vi "Controller Orbit Correction Algorithm.vi"(0 "FOFB Variables":T1, 1 "Corrector Kick Vector in":dbl[](array[numeric]), 2 "Beam Position Vector":dbl[](array[numeric]), 3 "Active?":bool, 5 "error in (no error)":errorcluster, 8 "Corrector Kick Vector Manual Setpoint in":dbl[](array[numeric])) -> (14 "Good value?":bool=TRUE, 15 "Corrector Kick Vector out":dbl[](array[numeric]), 19 "error out":errorcluster)   [LabVIEW 2011, in "Controller VIs.lvlib"]
doc: "Computes the correction algorithm to the selected BPM readings and returns the calculated corrector kick vector to be applied to the FOFB actuators."
uses:
  Controller VIs.lvlib
  Types Definitions/Type FOFB Variables.ctl
  Common VIs.lvlib
  Type Definitions.lvlib
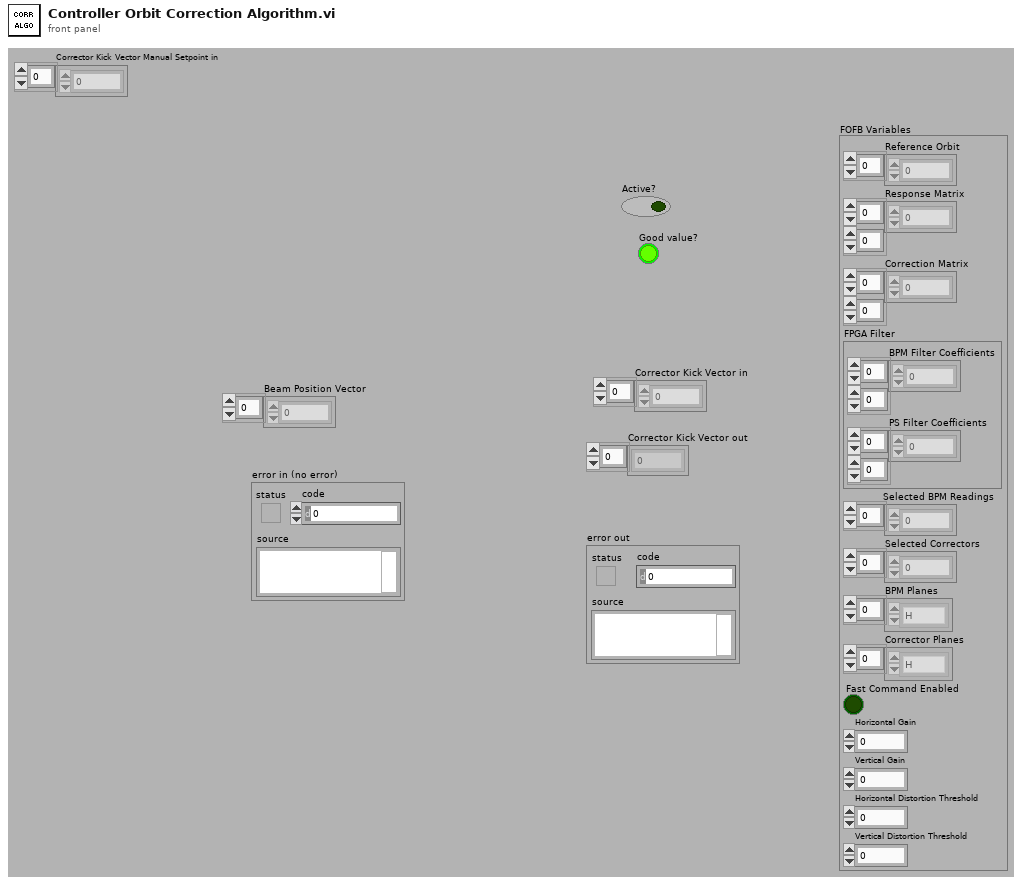
[diagram p1: front panel]
types:
  T1 = typedef "Type Definitions.lvlib/Type FOFB Variables.ctl" = cluster{"Reference Orbit":dbl[], "Response Matrix":dbl[][], "Correction Matrix":dbl[][], "FPGA Filter":cluster{"BPM Filter Coefficients":dbl[][], "PS Filter Coefficients":dbl[][]}, "Selected BPM Readings":u32[], "Selected Correctors":u32[], "BPM Planes":enum8{"H", "V"}[], "Corrector Planes":enum8{"H", "V"}[], "Fast Command Enabled":bool, "Horizontal Gain":dbl, "Vertical Gain":dbl, "Horizontal Distortion Threshold":dbl, "Vertical Distortion Threshold":dbl}
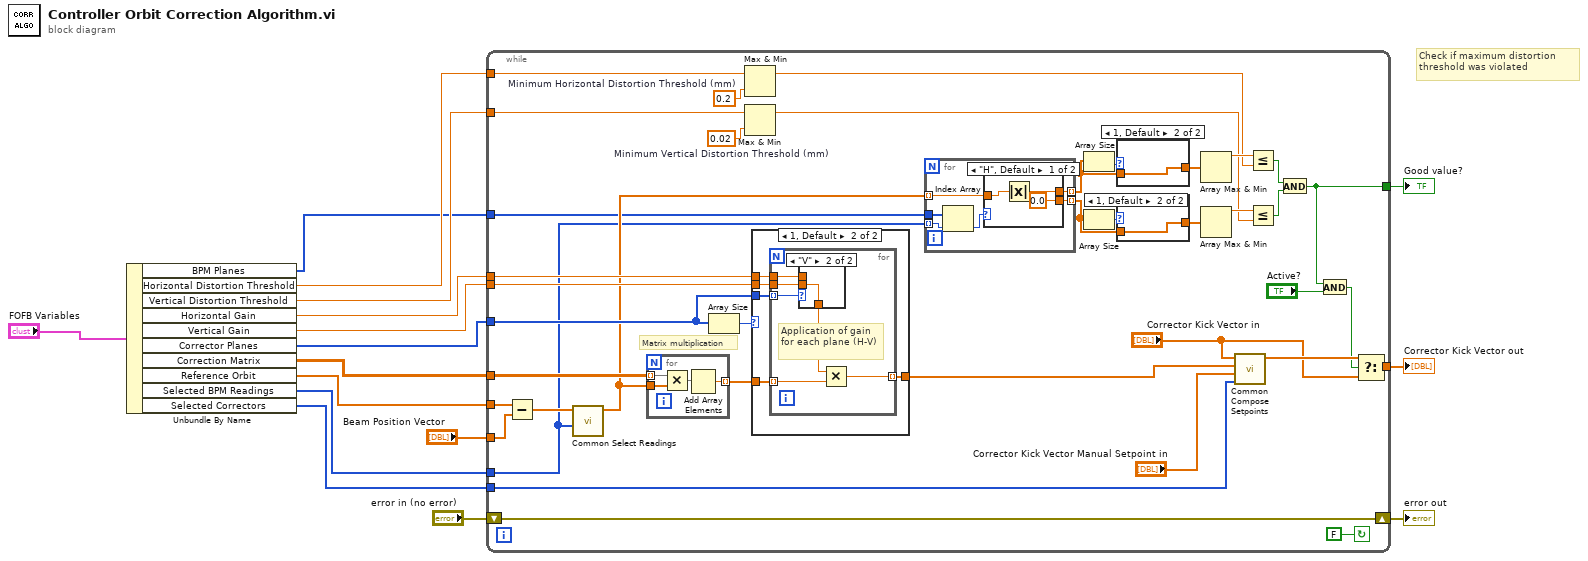
[diagram p0: block diagram]
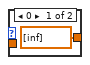
[diagram p2: hidden frame]
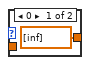
[diagram p3: hidden frame]
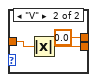
[diagram p4: hidden frame]
diagram:
  # "Check if maximum distortion threshold was violated"
  n1 = Unbundle By Name("FOFB Variables") -> ("BPM Planes"=w1:enum8{"H", "V"}[], "Horizontal Distortion Threshold"=w2:dbl, "Vertical Distortion Threshold"=w3:dbl, "Horizontal Gain"=w4:dbl, "Vertical Gain"=w5:dbl, "Corrector Planes"=w6:enum8{"H", "V"}[], "Correction Matrix"=w7:dbl[][], "Reference Orbit"=w12:dbl[], "Selected BPM Readings"=w9:u32[], "Selected Correctors"=w8:u32[])
  n2 = while {
    tunnel: w7 -> [w55]
    tunnel: w12 -> [w53]
    tunnel: "Beam Position Vector" -> [w52]
    shift-right: [w51] -> w14
    shift-left: "error in (no error)" -> [w51]
    tunnel: w6 -> [w49]
    tunnel: w9 -> [w17]
    tunnel: w8 -> [w33]
    tunnel: [w38] -> w11
    tunnel: [w45] -> w16
    tunnel: w5 -> [w40]
    tunnel: w4 -> [w39]
    tunnel: w2 -> [w31]
    tunnel: w3 -> [w28]
    tunnel: w1 -> [w25]
    stop <- FALSE continue-if-true
    w18 = 0.02  # Minimum Vertical Distortion Threshold (mm)
    w27 = 0.2  # Minimum Horizontal Distortion Threshold (mm)
    # "Matrix multiplication"
    n3 = Subtract(x=w53, y=w52) -> (x-y=w48:dbl[])
    n4 = call "Common Select Readings.vi"("Selected Readings"=w17, "Readings"=w48) -> ("Readings Subset"=w26:dbl[])  [unwired: 9 in]
    n5 = for {
      tunnel: w26 -> [w75]
      tunnel: w55 -> [w74] mode=indexing
      tunnel: [w72] -> w47 mode=indexing
      n6 = Multiply(x=w74, y=w75) -> (x*y=w73:dbl[])
      n7 = Add Array Elements(numeric array=w73) -> (sum=w72:dbl)
    }
    n8 = Array Size(array=w49) -> (size(s)=w50:i32)
    n9 = Max & Min(x=w31, y=w27) -> (max(x,y)=w30:dbl)  [unwired: 1 out]
    n10 = Max & Min(x=w28, y=w18) -> (max(x,y)=w29:dbl)  [unwired: 1 out]
    n11 = case shown="1, Default" w50 {
      tunnel: w47 -> [w76 w81]
      tunnel: [w76 w80] -> w43
      tunnel: w49 -> [_ w79]
      tunnel: w39 -> [_ w78]
      tunnel: w40 -> [_ w77]
      frame 0 {
      }
      frame 1, Default {
        n12 = for {
          tunnel: w81 -> [w86] mode=indexing
          tunnel: [w87] -> w80 mode=indexing
          tunnel: w79 -> [w85] mode=indexing
          tunnel: w78 -> [w83]
          tunnel: w77 -> [w82]
          # "Application of gain for each plane (H-V)"
          n13 = case shown="\"V\"" w85 {
            tunnel: [w88 w89] -> w84
            tunnel: w83 -> [w88 _]
            tunnel: w82 -> [_ w89]
            frame "H", Default {
            }
            frame "V" {
            }
          }
          n14 = Multiply(x=w84, y=w86) -> (x*y=w87:dbl)
        }
      }
    }
    n15 = for {
      tunnel: w26 -> [w65] mode=indexing
      tunnel: [w64] -> w21 mode=indexing
      tunnel: [w63] -> w20 mode=indexing
      tunnel: w25 -> [w62]
      tunnel: w17 -> [w61] mode=indexing
      n16 = Index Array(array=w62, index=w61) -> (element=w60:enum8{"H", "V"})
      n17 = case shown="\"H\", Default" w60 {
        tunnel: w65 -> [w68 w71]
        tunnel: [w67 0.0] -> w64
        tunnel: [0.0 w70] -> w63
        frame "H", Default {
          n18 = Absolute Value(x=w68) -> (abs(x)=w67:dbl)
        }
        frame "V" {
          n19 = Absolute Value(x=w71) -> (abs(x)=w70:dbl)
        }
      }
    }
    n20 = Array Size(array=w21) -> (size(s)=w23:i32)
    n21 = Array Size(array=w20) -> (size(s)=w19:i32)
    n22 = case shown="1, Default" w23 {
      tunnel: [dbl[] [inf] w57] -> w22
      tunnel: w21 -> [_ w57]
      frame 0 {
      }
      frame 1, Default {
      }
    }
    n23 = case shown="1, Default" w19 {
      tunnel: w20 -> [_ w59]
      tunnel: [dbl[] [inf] w59] -> w24
      frame 0 {
      }
      frame 1, Default {
      }
    }
    n24 = Array Max & Min(array=w22) -> (max value=w37:dbl)  [unwired: 3 out]
    n25 = Array Max & Min(array=w24) -> (max value=w36:dbl)  [unwired: 3 out]
    n26 = call "Common Compose Setpoints.vi"("Selected Correctors"=w33, "Corrector Kick Vector Manual Setpoint in"="Corrector Kick Vector Manual Setpoint in", "Corrector Kick Deltas Subset"=w43, "Corrector Kick Vector in"="Corrector Kick Vector in") -> ("Corrector Kicks"=w46:dbl[])  [unwired: 7 in]
    n27 = Less Or Equal?(x=w37, y=w30) -> (x <= y?=w35:bool)
    n28 = Less Or Equal?(x=w36, y=w29) -> (x <= y?=w34:bool)
    n29 = And(x=w35, y=w34) -> (x .and. y?=w38:bool)
    n30 = And(x=w38, y="Active?") -> (x .and. y?=w42:bool)
    n31 = Select(t=w46, s=w42, f="Corrector Kick Vector in") -> (s? t:f=w45:dbl[])
  }
  "error out" <- w14
  "Corrector Kick Vector out" <- w16
  "Good value?" <- w11
